vi "Motic Is Connected.vi"(8 "error in (no error)":errorcluster, 11 "camera":i32) -> (0 "error out":errorcluster, 2 "is connected?":bool, 3 "camera out":i32)   [LabVIEW 2012, in "MoticApi.lvlib"]
doc: "MOTICAPI bool Motic_IsConnected(MUCam_Handle camera);"
uses:
  MoticApi.lvlib
  MoticApi.dll
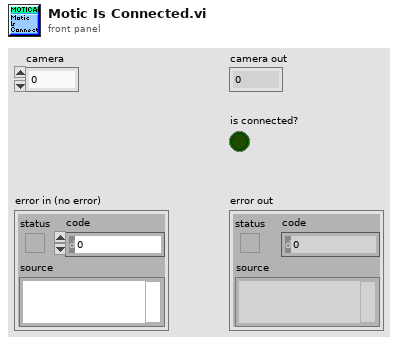
[diagram p1: front panel]
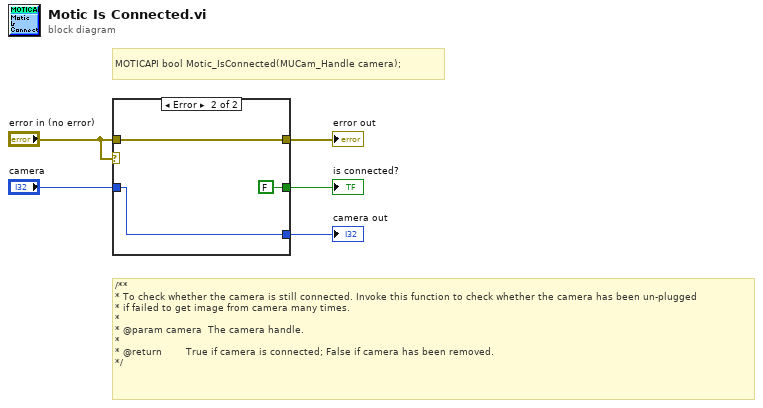
[diagram p0: block diagram]
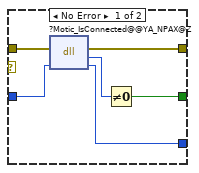
[diagram p2: hidden frame]
diagram:
  # "/**\n* To check whether the camera is still connected. Invoke this function to check whether the camera has been un-plugged\n* if failed to get image from camera many times.\n*\n* @param camera  The camera handle.\n*\n* @return        True if camera is connected; False if camera has been removed.\n*/"
  # "MOTICAPI bool Motic_IsConnected(MUCam_Handle camera);"
  n1 = case shown="Error" "error in (no error)" {
    tunnel: [w11 FALSE] -> w5
    tunnel: "camera" -> [w9 w12]
    tunnel: [w8 w12] -> w3
    tunnel: "error in (no error)" -> [w7 w14]
    tunnel: [w6 w14] -> w2
    frame No Error {
      n2 = dll-call lib="C:/Users/TTS-Digital/Desktop/MoticApi/MoticApi_git/MoticApi/MoticApi.*" fn="?Motic_IsConnected@@YA_NPAX@Z"(error in=w7, "camera"=w9) -> (error out=w6:errorcluster, w10:u8, "camera"=w8:i32)  [unwired: 2 in, 1 out]
      n3 = Not Equal To 0?(x=w10) -> (x != 0?=w11:bool)
    }
    frame Error {
    }
  }
  "is connected?" <- w5
  "camera out" <- w3
  "error out" <- w2
